vi "File.Rotate.Read Config with Dialog Option.vi"(8 "error in (no error)":errorcluster, 9 "Dialog":bool, 10 "Config File":path, 11 "File.Rotate in":refnum<class "File.Rotate.lvclass">) -> (0 "error out":errorcluster, 1 "Saved":bool, 2 "Tasks":T1[](array[typedef]), 3 "File.Rotate out":refnum<class "File.Rotate.lvclass">)   [LabVIEW 2024, in "KATE_Lib.lvlib" / "File Utils.lvlib" / "File.Rotate.lvclass"]
uses:
  File.Rotate.lvclass
  File.Rotate.Rotation Task Item.ctl
  File.Rotate.lvclass/File.Rotate.ctl
  File Utils.lvlib
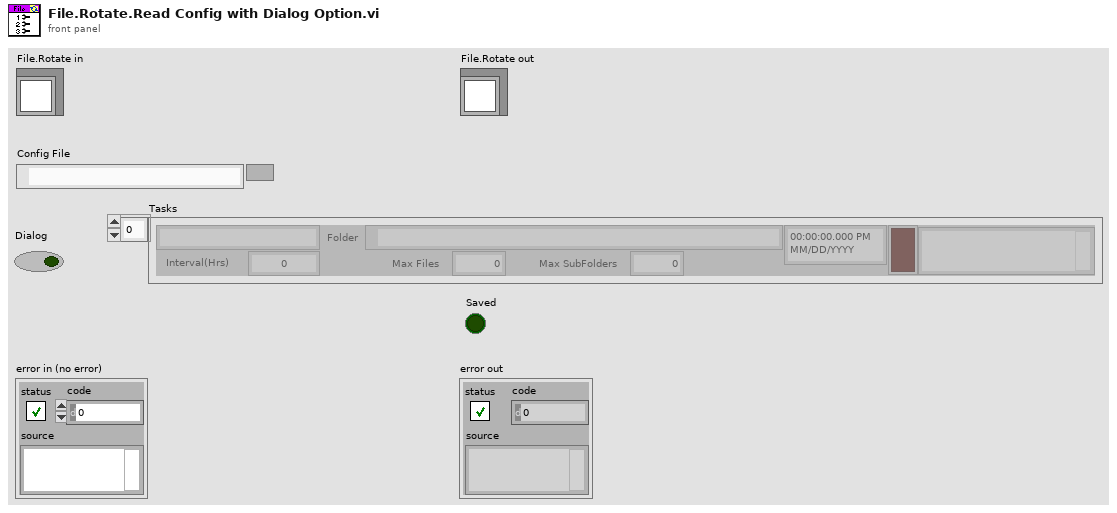
[diagram p1: front panel]
types:
  T1 = typedef "KATE_Lib.lvlib/File Utils.lvlib/File.Rotate.lvclass/File.Rotate.Rotation Task Item.ctl" = cluster{"Name":string, "Interval":dbl, "Folder":path, "Max Files":i32, "Max SubFolders":i32, "LastRotate":timestamp, "Error":bool, "Status":string}
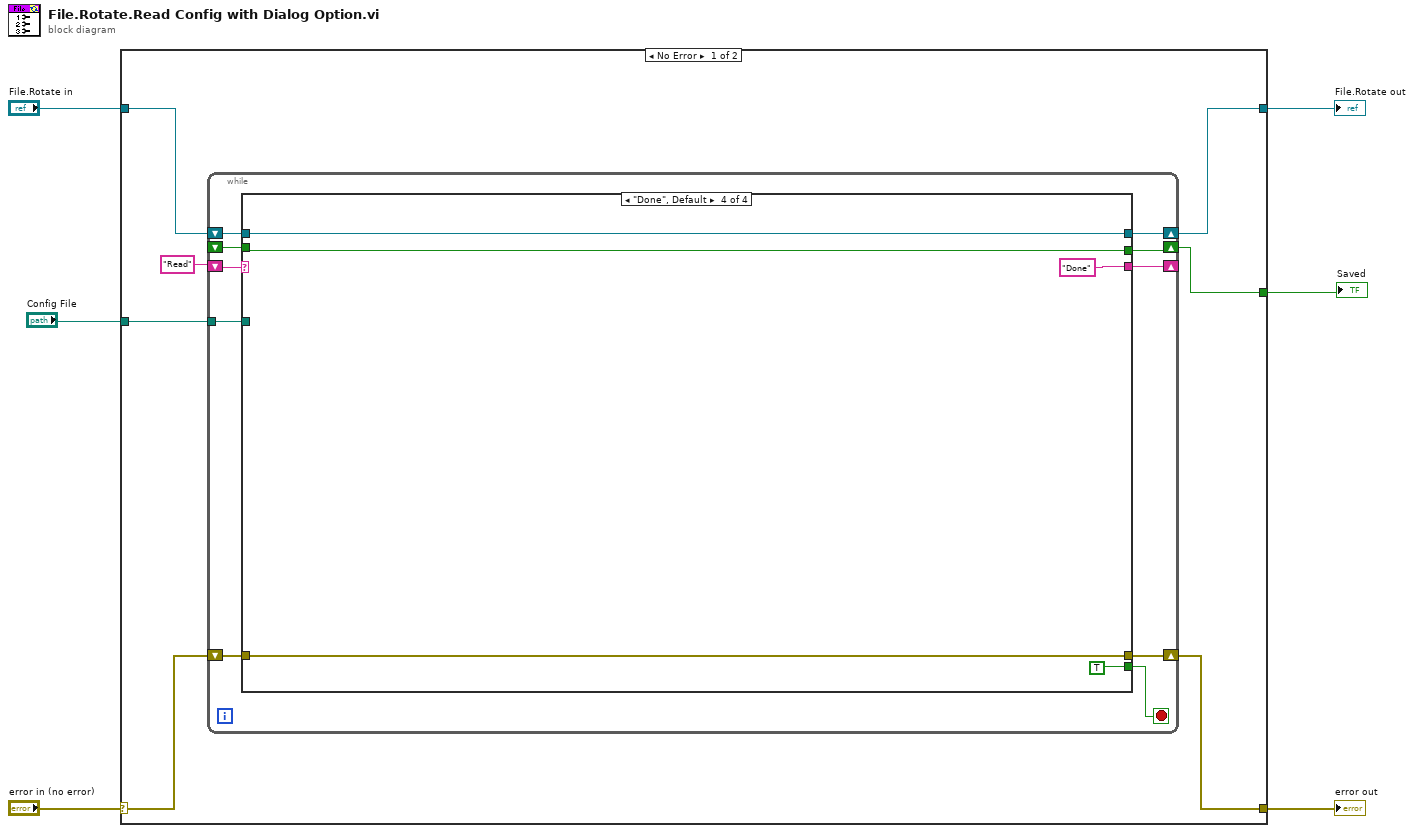
[diagram p0: block diagram]
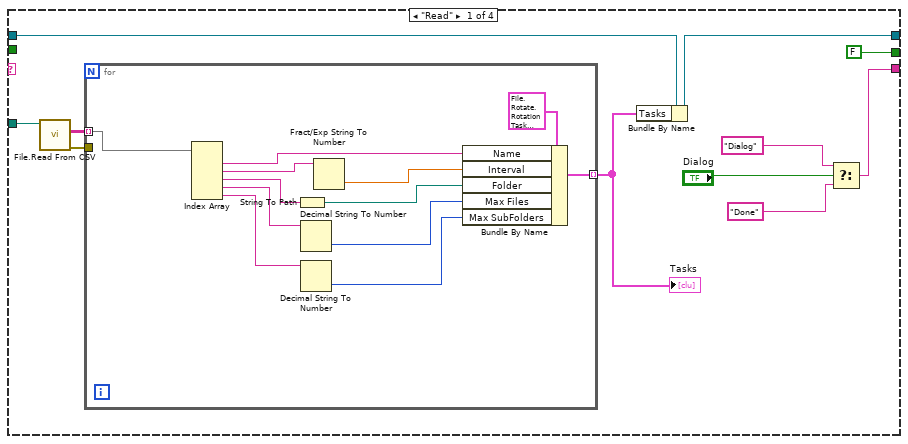
[diagram p2: hidden frame]
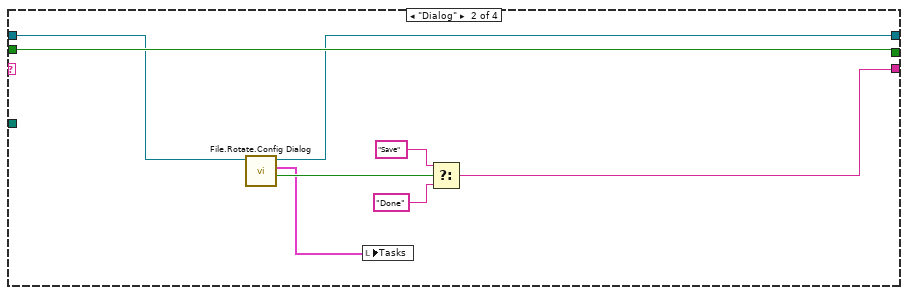
[diagram p3: hidden frame]
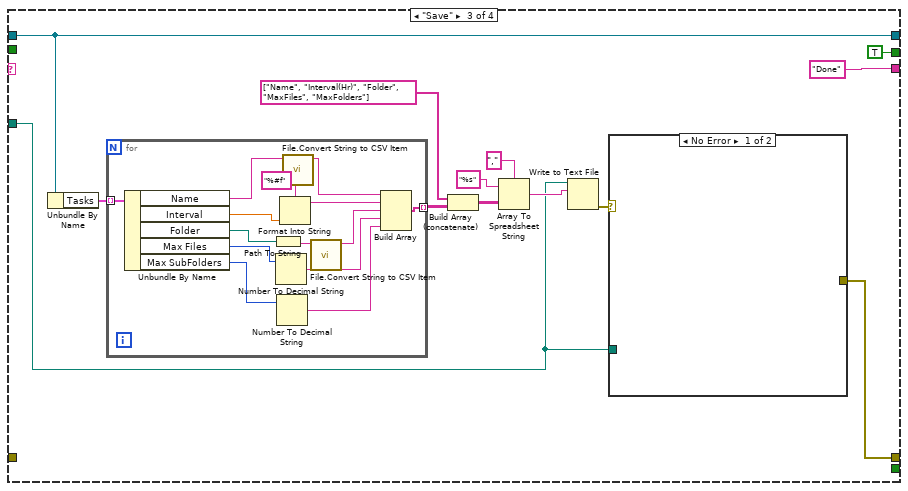
[diagram p4: hidden frame]
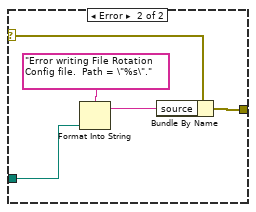
[diagram p5: hidden frame]
diagram:
  n1 = case shown="No Error" "error in (no error)" {
    selector: "error in (no error)" -> [w11 w93]
    tunnel: [w10 w93] -> w5
    tunnel: [w9 w92] -> w3
    tunnel: "File.Rotate in" -> [w8 w92]
    tunnel: "Config File" -> [w12 _]
    tunnel: [w7 _] -> w1
    frame No Error {
      n2 = while {
        tunnel: w12 -> [w23]
        shift-right: [w21] -> w9
        shift-left: w8 -> [w22]
        shift-right: [w18] -> _
        shift-left: "Read" -> [w19]
        shift-right: [w17] -> w10
        shift-left: w11 -> [w20]
        shift-right: [w14] -> w7
        shift-left: _ -> [w15]
        stop <- w16 stop-if-true
        n3 = case shown="\"Done\", Default" w19 {
          tunnel: w23 -> [w34 _ w57 _]
          tunnel: w22 -> [w32 w53 w67 w91]
          tunnel: [w31 w52 w67 w91] -> w21
          tunnel: w20 -> [_ _ _ w89]
          tunnel: [w26 w48 "Done" "Done"] -> w18
          tunnel: [_ _ w56 w89] -> w17
          tunnel: [_ _ _ TRUE] -> w16
          tunnel: w15 -> [_ w54 _ w87]
          tunnel: [FALSE w54 TRUE w87] -> w14
          frame "Read" {
            n4 = call "File.Read From CSV.vi"("File"=w34) -> ("error out"=w24:errorcluster, "Data"=w33:string[][])  [unwired: 8 in, 1 out]
            n5 = for {
              tunnel: w33 -> [w41] mode=indexing
              tunnel: [w43] -> w30 mode=indexing
              tunnel: w24 -> [_]
              n6 = Index Array(array=w41) -> (element #1=w45:string, element #2=w44:string, element #3=w39:string, element #4=w38:string, element #5=w37:string)  [unwired: 5 in]
              n7 = String To Path(string=w39) -> (path=w40:path)
              n8 = Decimal String To Number(string=w38) -> (number=w36:i32)  [unwired: 2 in, 1 out]
              n9 = Decimal String To Number(string=w37) -> (number=w35:i32)  [unwired: 2 in, 1 out]
              n10 = Fract/Exp String To Number(string=w44) -> (number=w42:dbl)  [unwired: 3 in, 1 out]
              n11 = Bundle By Name(cluster=T1 {"Name"="", "Interval"=12.0, "Folder"=path "", "Max Files"=1000, "Max SubFolders"=1000, "LastRotate"=timestamp(0 s since 1904-01-01), "Error"=FALSE, "Status"=""} ("SyncItem"), "Name"=w45, "Interval"=w42, "Folder"=w40, "Max Files"=w36, "Max SubFolders"=w35) -> (w43:T1)
            }
            "Tasks" <- w30
            n12 = Bundle By Name(cluster=w32, "Tasks"=w30) -> (w31:refnum<class "File.Rotate.lvclass">)
            n13 = Select(t="Dialog", s="Dialog", f="Done") -> (s? t:f=w26:string)
          }
          frame "Dialog" {
            n14 = call "File.Rotate.Config Dialog.vi"("File.Rotate in"=w53) -> ("OK"=w51:bool, "Rotation Config"=w47:T1[], "File.Rotate out"=w52:refnum<class "File.Rotate.lvclass">)  [unwired: 7 in, 1 out]
            n15 = local write "Tasks"(w47) -> ()
            n16 = Select(t="Save", s=w51, f="Done") -> (s? t:f=w48:string)
          }
          frame "Save" {
            n17 = Unbundle By Name(w67) -> ("Tasks"=w65:T1[])
            n18 = for {
              tunnel: w65 -> [w86] mode=indexing
              tunnel: [w85] -> w63 mode=indexing
              n19 = Unbundle By Name(w86) -> ("Name"=w84:string, "Interval"=w82:dbl, "Folder"=w79:path, "Max Files"=w76:i32, "Max SubFolders"=w75:i32)
              n20 = Path To String(path=w79) -> (string=w78:string)
              n21 = Number To Decimal String(number=w76) -> (decimal integer string=w74:string)  [unwired: 1 in]
              n22 = Number To Decimal String(number=w75) -> (decimal integer string=w73:string)  [unwired: 1 in]
              n23 = Format Into String(format string="%#f", w82) -> (resulting string=w81:string)  [unwired: 2 in, 1 out]
              n24 = call "File.Convert String to CSV Item.vi"("String"=w84) -> ("String Out"=w83:string)  [unwired: 10 in]
              n25 = call "File.Convert String to CSV Item.vi"("String"=w78) -> ("String Out"=w77:string)  [unwired: 10 in]
              n26 = Build Array(w83, w81, w77, w74, w73) -> (w85:string[])
            }
            n27 = Build Array (concatenate)(string[] ["Name", "Interval(Hr)", "Folder", "MaxFiles", "MaxFolders"], w63) -> (w62:string[][])
            n28 = Array To Spreadsheet String(delimiter (Tab)=",", array=w62, 3:"%s" ("format string")) -> (spreadsheet string=w59:string)
            n29 = Write to Text File(file (use dialog)=w57, text=w59) -> (error out=w58:errorcluster)  [unwired: 2 in, 2 out]
            n30 = case shown="No Error" w58 {
              selector: w58 -> [_ w72]
              tunnel: w57 -> [_ w69]
              tunnel: [_ w71] -> w56
              frame No Error {
              }
              frame Error {
                n31 = Format Into String(format string="Error writing File Rotation Config file.  Path = \"%s\".", w69) -> (resulting string=w68:string)  [unwired: 2 in, 1 out]
                n32 = Bundle By Name(cluster=w72, "source"=w68) -> (w71:errorcluster)
              }
            }
          }
          frame "Done", Default {
          }
        }
      }
    }
    frame Error {
    }
  }
  "error out" <- w5
  "File.Rotate out" <- w3
  "Saved" <- w1
